vi "Read Snake DVR.vi"(8 "error in (no error)":errorcluster, 10 "data value reference":refnum<data-value>) -> (0 "error out":errorcluster, 2 "Snake":refnum<class "Snake.lvclass">)   [LabVIEW 2021, in "Board Game.lvclass"]
uses:
  Board Game.lvclass
  Snake_class/Snake.lvclass
  Board Game.lvclass/Board Game.ctl
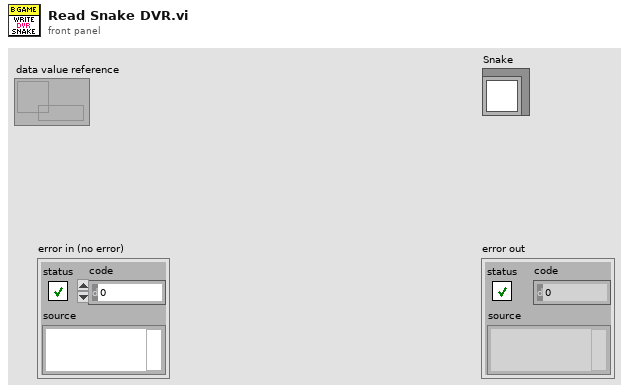
[diagram p1: front panel]
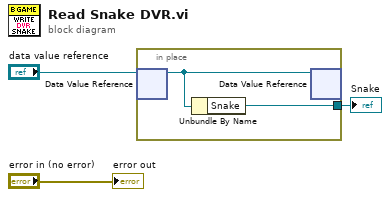
[diagram p0: block diagram]
diagram:
  n1 = in-place {
    in-place-border: [w4] -> w1
    n2 = in-place-dvr #1("data value reference") -> (w5:refnum<class "Board Game.lvclass">)  [unwired: 1 out]
    n3 = Unbundle By Name(w5) -> ("Snake"=w4:refnum<class "Snake.lvclass">)
    n4 = in-place-dvr #1(w5) -> ()  [unwired: 2 out]
  }
  "Snake" <- w1
  "error out" <- "error in (no error)"
